vi "getType.vi"(8 "error in (no error)":errorcluster, 11 "Xcite in":refnum<class "Xcite.lvclass">) -> (0 "error out":errorcluster, 2 "type":u16(ring)=65535 items=["XC_120PC"=0, "XC_exacte"=1, "XC_120LED"=2, "XC_110LED"=3, "XC_mini"=4, "XC_XYLIS"=5, "XC_XR210"=6, "XC_LED1"=7, "XC_XT600"=8, "XC_XT900"=9, "Any"=65535], 3 "Xcite out":refnum<class "Xcite.lvclass">)   [LabVIEW 2019, in "Xcite.lvclass"]
doc: "Gets the XCite device type."
uses:
  Xcite.lvclass
  Xcite.lvclass/Xcite.ctl
  etc.xcite/XCite.lvlib
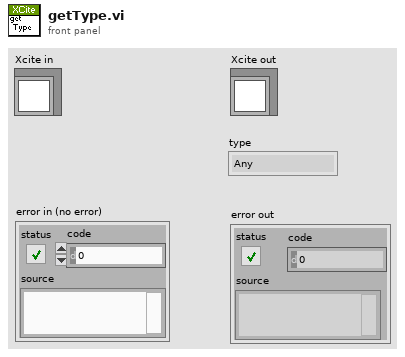
[diagram p1: front panel]
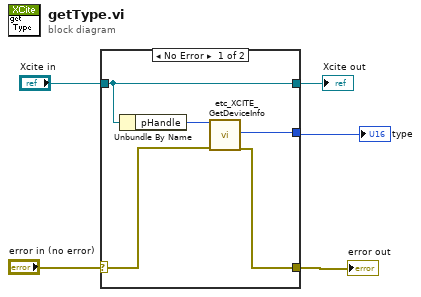
[diagram p0: block diagram]
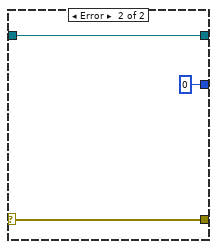
[diagram p2: hidden frame]
diagram:
  n1 = case shown="No Error" "error in (no error)" {
    selector: "error in (no error)" -> [w10 w13]
    tunnel: [w9 w13] -> w4
    tunnel: "Xcite in" -> [w7 w11]
    tunnel: [w8 0 ("type")] -> w1
    tunnel: [w7 w11] -> w2
    frame No Error {
      n2 = Unbundle By Name(w7) -> ("pHandle"=w6:u64)
      n3 = call "etc_XCITE_GetDeviceInfo.vi"("h"=w6, "error in (no error)"=w10) -> ("type"=w8:i32, "error out"=w9:errorcluster)  [unwired: 12 in, 4 out]
    }
    frame Error {
    }
  }
  "Xcite out" <- w2
  "error out" <- w4
  "type" <- w1
